vi "valve_controll_vi.vi"(10 "Value (0)":u8) -> ()   [LabVIEW 2011]
uses:
  <vilib>/LabVIEW Interface for Arduino/Type Defs/Pin Mode.ctl
  <vilib>/LabVIEW Interface for Arduino/LabVIEW Interface for Arduino.lvlib
panel:
  in  "VISA resource":refnum<visa-resource-name>
  in  "Digital I/O Pin":u8
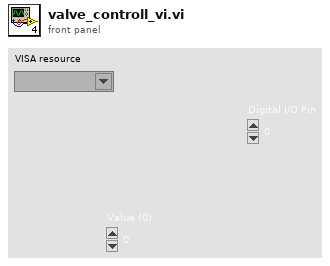
[diagram p1: front panel]
types:
  T1 = typedef "LabVIEW Interface for Arduino.lvlib/Pin Mode.ctl" = enum8{"Input", "Output"}
  T2 = typedef "LabVIEW Interface for Arduino.lvlib/Arduino Resource.ctl" = cluster{"VISA resource":refnum<visa-resource-name>, "Board Type":T3, "Connection Type":enum8{"USB / Serial"}, "Bytes Per Packet (15)":u8}
  T3 = typedef "LabVIEW Interface for Arduino.lvlib/Board Type.ctl" = enum16{"Uno", "Dimuelanove w/Atmega 328", "Mega 2560"}
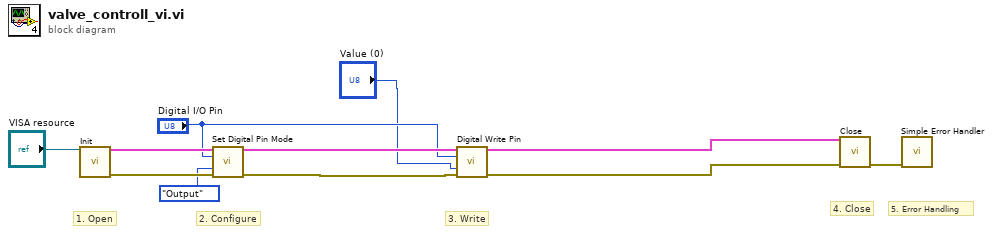
[diagram p0: block diagram]
diagram:
  # "3. Write"
  # "5. Error Handling"
  # "4. Close"
  # "2. Configure"
  # "1. Open"
  n1 = call <vilib>:"Init.vi"("VISA resource"="VISA resource") -> ("Arduino Resource"=w8:T2, "error out"=w7:errorcluster)  [unwired: 17 in]
  n2 = call <vilib>:"Set Digital Pin Mode.vi"("Arduino Resource"=w8, "Digital I/O Pin"="Digital I/O Pin", "Pin Mode (Input)"=Pin_Mode."Output", "error in"=w7) -> ("Arduino Resource"=w6:T2, "error out"=w5:errorcluster)  [unwired: 10 in]
  n3 = call <vilib>:"Digital Write Pin.vi"("Arduino Resource"=w6, "Digital I/O Pin (0)"="Digital I/O Pin", "Value (0)"="Value (0)", "error in"=w5) -> ("Arduino Resource"=w10:T2, "error out"=w9:errorcluster)  [unwired: 10 in]
  n4 = call <vilib>:"Close.vi"("Arduino Resource"=w10, "error in"=w9) -> ("error out"=w11:errorcluster)  [unwired: 13 in]
  n5 = call <vilib>:"Simple Error Handler.vi"("error in (no error)"=w11) -> ()  [unwired: 4 in, 5 out]
